vi "Update AO Sweep Status.vi"(8 "error in (no error)":errorcluster, 10 "Channels: AO.Sweeping?":bool[](array[boolean]), 11 "Generator in":refnum<class "Generator.lvclass">) -> (0 "error out":errorcluster, 3 "Generator out":refnum<class "Generator.lvclass">)   [LabVIEW 2019, in "Generator.lvclass"]
uses:
  Generator.lvclass
  Generator.lvclass/Generator.ctl
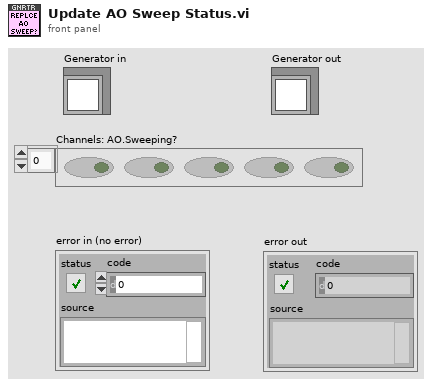
[diagram p1: front panel]
types:
  T1 = typedef "Generator.lvclass/AO.Channel--Cluster--Array.ctl" = T2[]
  T2 = typedef "Generator.lvclass/AO.Channel--Cluster.ctl" = cluster{"Enable?":bool, "Channel":i32, "Amplitude":dbl, "Offset":dbl, "Frequency":dbl, "Phase":dbl, "Function":T3, "Sweeping?":bool, "Limit AC?":bool, "Limit DC?":bool, "Duty Cycle?":bool, "Duty Cycle":dbl}
  T3 = typedef "Generator.lvclass/AO.Channel.Function--Enum.ctl" = enum16{"sine", "square", "triangle", "saw"}
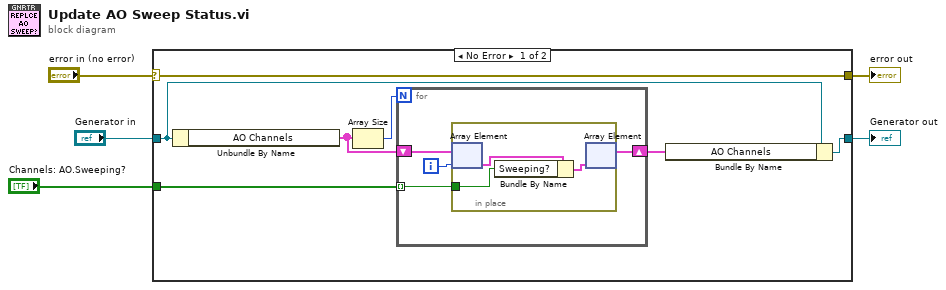
[diagram p0: block diagram]
diagram:
  n1 = case shown="No Error" "error in (no error)" {
    selector: "error in (no error)" -> [w6 w21]
    tunnel: "Channels: AO.Sweeping?" -> [w12 _]
    tunnel: "Generator in" -> [w11 w20]
    tunnel: [w6 w21] -> w2
    tunnel: [w9 w20] -> w1
    frame No Error {
      n2 = Unbundle By Name(w11) -> ("AO Channels"=w7:T1)
      n3 = Array Size(array=w7) -> (size(s)=w8:i32)
      n4 = for {
        N: w8 -> [_]
        tunnel: w12 -> [w16] mode=indexing
        shift-right: [w13] -> w10
        shift-left: w7 -> [w15]
        i -> [w14]
        n5 = in-place {
          in-place-border: w16 -> [w19]
          n6 = in-place-array #1(w15, w14) -> (w18:T2)
          n7 = Bundle By Name(cluster=w18, "Sweeping?"=w19) -> (w17:T2)
          n8 = in-place-array #1(w17) -> (w13:T1)  [unwired: 1 out]
        }
      }
      n9 = Bundle By Name(cluster=w11, "AO Channels"=w10) -> (w9:refnum<class "Generator.lvclass">)
    }
    frame Error {
    }
  }
  "Generator out" <- w1
  "error out" <- w2
